vi "merFISH_define_buffer_probe_lists.vi"(4 "error in":errorcluster, 5 "Start acquisition":bool, 6 "Probe Refnum":refnum<vi>, 7 "Buffer Refnum":refnum<vi>) -> (0 "error out":errorcluster, 3 "Next task":T1)   [LabVIEW 2015]
uses:
  CONTROLS/Q_main_element.ctl
panel:
  in  "Remove probe":bool
  in  "Remove buffer":bool
  in  "stop":bool
  in  "merFISH probe":string
  in  "Valve #":i32
  in  "Add probe":bool
  in  "Buffer":string
  in  "Probe list":i32(listbox)=1
  in  "Buffer list":i32(listbox)=3
  in  "Valve #":i32
  in  "Add buffer":bool
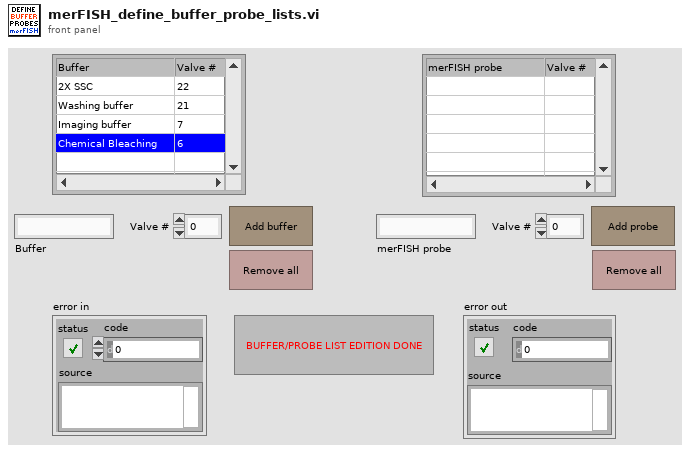
[diagram p1: front panel]
types:
  T1 = typedef "Q_main_element.ctl" = cluster{"variant":variant, "Instruction":enum16{"Main_idle", "Main_initialize", "Main_initialize_TDMS", "Main_initialize_Queue", "Main_error", "Main_DAQ_initialization_results", "Main_ASI_initialization_results", "Main_Piezo_initialization_results", "Main_Valve_initialization_results", "Main_Pump_initialization_results", "Main_CAMERA_initialization_results", "Main_FPGA_initialization_results", "Main_DAQ_error", "Main_ASI_error", "Main_Piezo_error", "Main_CAMERA_error", "Main_Valve_error", "Main_Pump_error", "Main_FPGA_error", "Main_start_acquiring", "Main_not_acquiring", "Main_acquiring", "Main_stop_acquiring", "Main_change_exposure", "Main_change_z_scan_parameters", "Main_define_ROI", "Main_define_mosaic", "Main_read_kinetic_time", "Main_cooler", "Main_read_temperature", "Main_save_XY", "Main_load_XY", "Main_discard_XY", "Main_move_to_XY", "Main_measure_QPD", "Main_autofocus_calibration", "Main_autofocus_initialization", "Main_autofocus_stop", "Main_save_PID", "Main_change_H_valve_position", "Main_two_way_valve", "Main_save_movie", "Main_init_single_scan", "Main_single_scan", "Main_stop_single_scan", "Main_merFISH_illumination_parameters", "Main_merFISH_buffer_probe_list", "Main_merFISH_injections_procedure", "Main_merFISH_save_setpoint", "Main_merFISH_DAPI_parameters", "Main_merFISH_Brightfield_parameters", "Main_merFISH_save_embryo_ROI", "Main_merFISH_init", "Main_merFISH_resume", "Main_merFISH_start_autofocus", "Main_merFISH_open_close_valve_merFISH", "Main_merFISH_open_close_valve_photobleaching", "Main_merFISH_hybridization", "Main_merFISH_move_to_ROI", "Main_merFISH_wait_stabilization", "Main_merFISH_move_to_REF", "Main_merFISH_scan", "Main_merFISH_photobleaching_injection", "Main_merFISH_photobleaching", "Main_merFISH_send_email", "Main_merFISH_close", "Main_STOP"}}
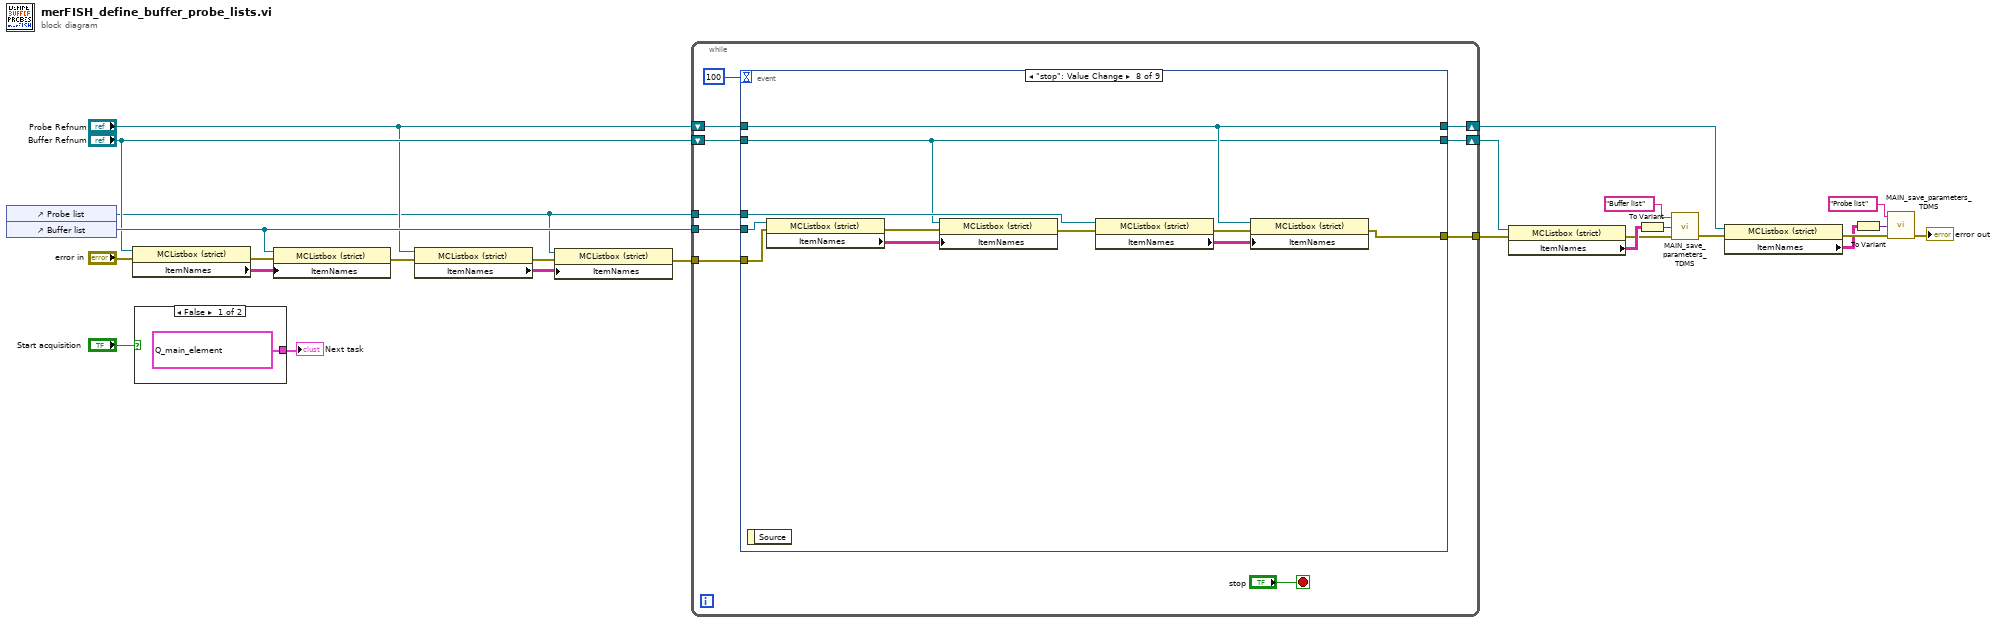
[diagram p0: block diagram]
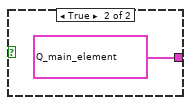
[diagram p2: hidden frame]
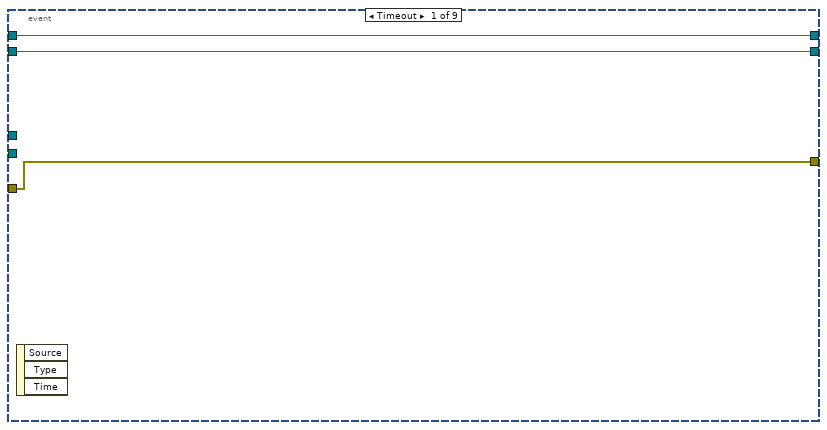
[diagram p3: hidden frame]
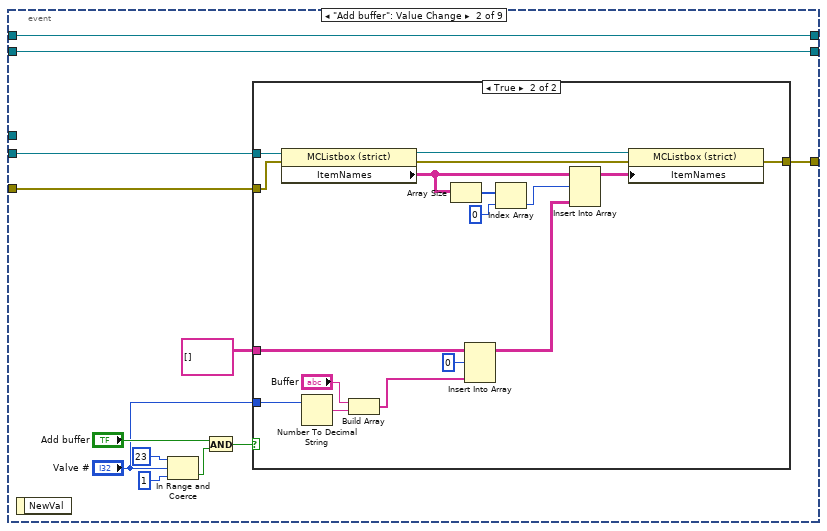
[diagram p4: hidden frame]
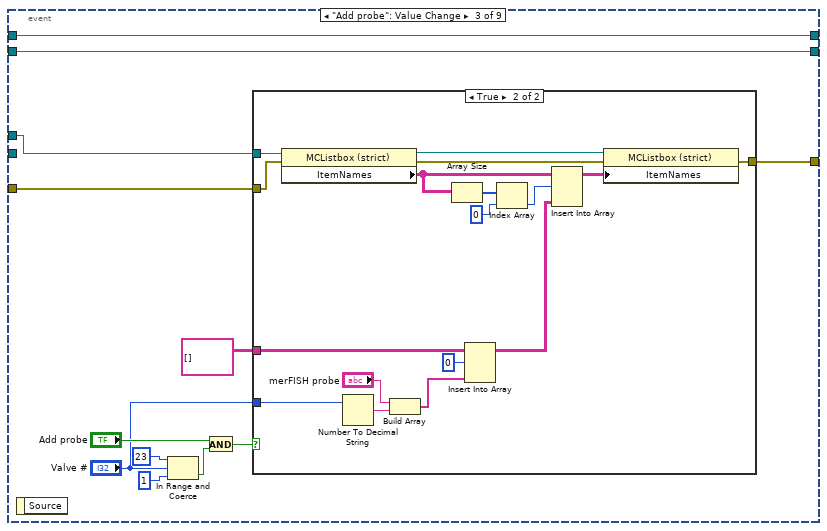
[diagram p6: hidden frame]
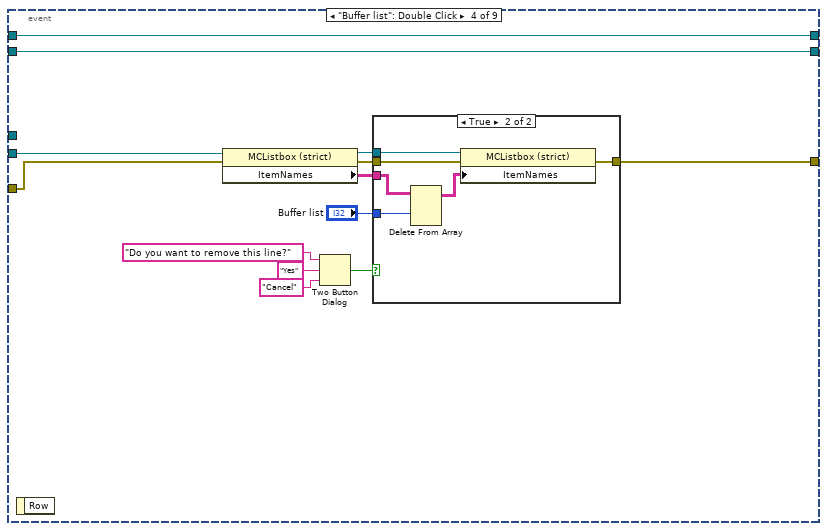
[diagram p8: hidden frame]
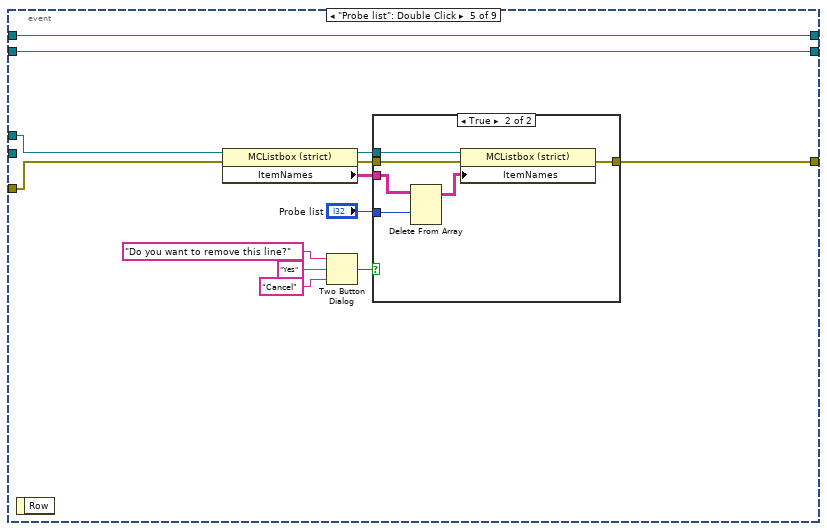
[diagram p10: hidden frame]
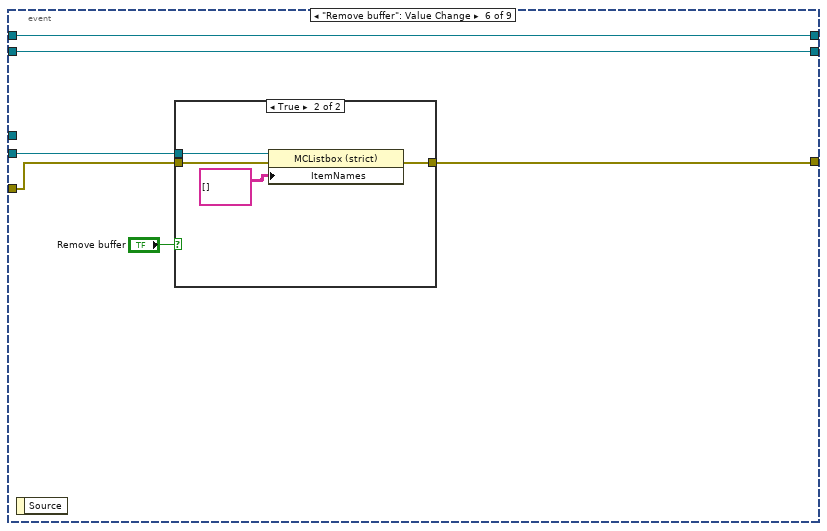
[diagram p12: hidden frame]
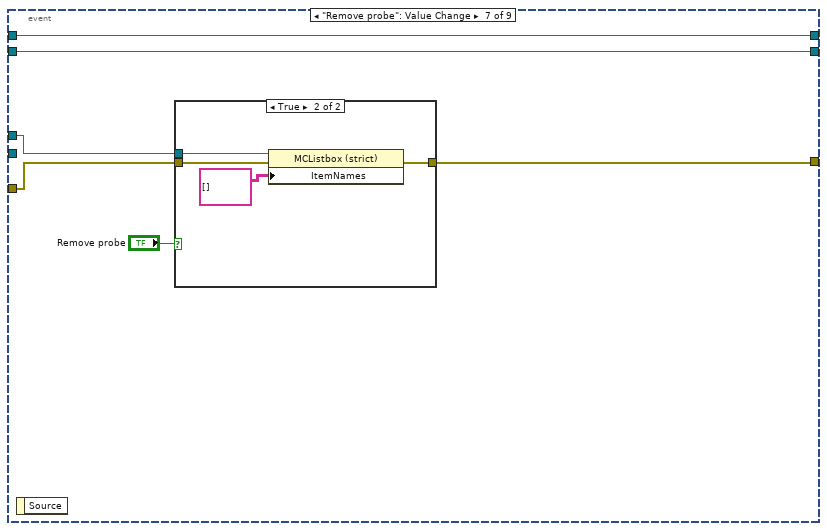
[diagram p14: hidden frame]
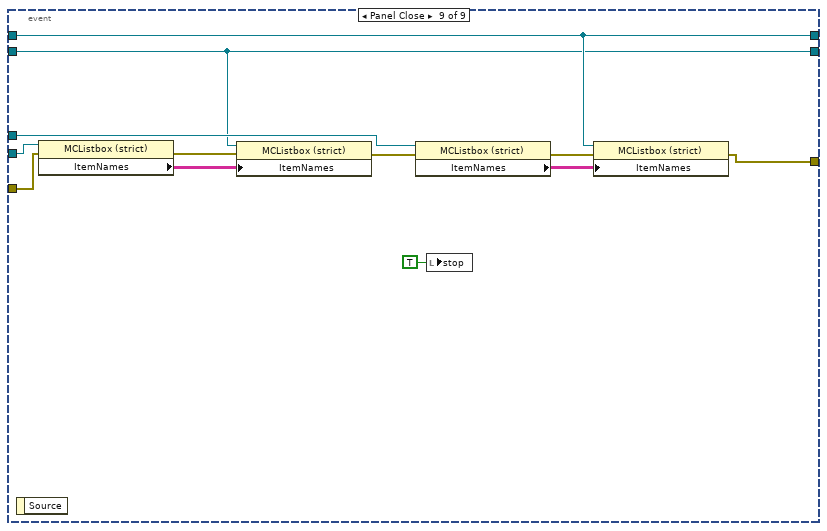
[diagram p16: hidden frame]
diagram:
  n1 = control-ref of="Probe list"() -> (w16:refnum<vi>)
  n2 = control-ref of="Buffer list"() -> (w26:refnum<vi>)
  n3 = property class="MCListbox (strict)"(reference="Buffer Refnum", error in="error in") -> (error out=w25:errorcluster, "ItemNames"=w23:string[][])  [unwired: 1 out]
  n4 = case shown="False" "Start acquisition" {
    tunnel: [T1 {"variant"=variant, "Instruction"=enum."Main_not_acquiring"} ("Q_main_element") T1 {"variant"=variant, "Instruction"=enum."Main_acquiring"} ("Q_main_element")] -> w1
    frame False {
    }
    frame True {
    }
  }
  "Next task" <- w1
  n5 = property class="MCListbox (strict)"(reference=w26, error in=w25, "ItemNames"=w23) -> (error out=w20:errorcluster)  [unwired: 1 out]
  n6 = property class="MCListbox (strict)"(reference="Probe Refnum", error in=w20) -> (error out=w21:errorcluster, "ItemNames"=w22:string[][])  [unwired: 1 out]
  n7 = property class="MCListbox (strict)"(reference=w16, error in=w21, "ItemNames"=w22) -> (error out=w18:errorcluster)  [unwired: 1 out]
  n8 = while {
    tunnel: w26 -> [w37]
    tunnel: w16 -> [w36]
    tunnel: [w35] -> w8
    tunnel: w18 -> [w31]
    shift-right: [w30] -> w3
    shift-left: "Probe Refnum" -> [w33]
    shift-right: [w29] -> w4
    shift-left: "Buffer Refnum" -> [w32]
    stop <- "stop" stop-if-true
    n9 = event shown="[7] \"stop\": Value Change" {
      selector: _ -> [_ _ _ _ _ _ _ _ _]
      dyn-events: _ -> [_ _ _ _ _ _ _ _ _]
      timeout: 100 -> [_ _ _ _ _ _ _ _ _]
      tunnel: [w41 w47 w79 w110 w130 w145 w158 w170 w182] -> w35
      tunnel: w37 -> [_ w46 _ w106 _ w146 _ w169 w181]
      tunnel: w36 -> [_ _ w77 _ w125 _ w156 w173 w185]
      tunnel: w33 -> [w40 w43 w73 w103 w123 w143 w154 w165 w176]
      tunnel: w32 -> [w39 w42 w72 w102 w122 w142 w153 w164 w175]
      tunnel: w31 -> [w41 w44 w74 w104 w124 w144 w155 w168 w180]
      tunnel: [w40 w43 w73 w103 w123 w143 w154 w165 w176] -> w30
      tunnel: [w39 w42 w72 w102 w122 w142 w153 w164 w175] -> w29
      event Timeout {
        n10 = event-data() -> ()  [unwired: 1 in, 3 out]
      }
      event "Add buffer": Value Change {
        n11 = event-data() -> ()  [unwired: 1 in, 1 out]
        n12 = In Range and Coerce(upper limit=23, x="Valve #", lower limit=1) -> (In Range?=w51:bool)  [unwired: 1 out]
        n13 = And(x="Add buffer", y=w51) -> (x .and. y?=w49:bool)
        n14 = case shown="True" w49 {
          tunnel: w46 -> [_ w71]
          tunnel: string[][] [] ("Item Names") -> [_ w70]
          tunnel: "Valve #" -> [_ w69]
          tunnel: [w54 w59] -> w47
          tunnel: w44 -> [w54 w58]
          frame False {
          }
          frame True {
            n15 = property class="MCListbox (strict)"(reference=w71, error in=w58) -> (reference out=w55:refnum<vi>, error out=w56:errorcluster, "ItemNames"=w57:string[][])
            n16 = Number To Decimal String(number=w69) -> (decimal integer string=w67:string)  [unwired: 1 in]
            n17 = Build Array("Buffer", w67) -> (w65:string[])
            n18 = Array Size(array=w57) -> (size(s)=w64:i32[])
            n19 = Insert Into Array(array=w70, index (row)=0, new element=w65) -> (w62:string[][])  [unwired: 1 in]
            n20 = Index Array(array=w64, index=0) -> (element=w61:i32)
            n21 = Insert Into Array(array=w57, index (row)=w61, new element=w62) -> (w60:string[][])  [unwired: 1 in]
            n22 = property class="MCListbox (strict)"(reference=w55, error in=w56, "ItemNames"=w60) -> (error out=w59:errorcluster)  [unwired: 1 out]
          }
        }
      }
      event "Add probe": Value Change {
        n23 = event-data() -> ()  [unwired: 1 in, 1 out]
        n24 = In Range and Coerce(upper limit=23, x="Valve #", lower limit=1) -> (In Range?=w81:bool)  [unwired: 1 out]
        n25 = And(x="Add probe", y=w81) -> (x .and. y?=w80:bool)
        n26 = case shown="True" w80 {
          tunnel: w77 -> [_ w101]
          tunnel: string[][] [] ("Item Names") -> [_ w100]
          tunnel: "Valve #" -> [_ w99]
          tunnel: [w84 w98] -> w79
          tunnel: w74 -> [w84 w88]
          frame False {
          }
          frame True {
            n27 = property class="MCListbox (strict)"(reference=w101, error in=w88) -> (reference out=w87:refnum<vi>, error out=w86:errorcluster, "ItemNames"=w85:string[][])
            n28 = Number To Decimal String(number=w99) -> (decimal integer string=w96:string)  [unwired: 1 in]
            n29 = Build Array("merFISH probe", w96) -> (w95:string[])
            n30 = Array Size(array=w85) -> (size(s)=w94:i32[])
            n31 = Insert Into Array(array=w100, index (row)=0, new element=w95) -> (w91:string[][])  [unwired: 1 in]
            n32 = Index Array(array=w94, index=0) -> (element=w92:i32)
            n33 = Insert Into Array(array=w85, index (row)=w92, new element=w91) -> (w90:string[][])  [unwired: 1 in]
            n34 = property class="MCListbox (strict)"(reference=w87, error in=w86, "ItemNames"=w90) -> (error out=w98:errorcluster)  [unwired: 1 out]
          }
        }
      }
      event "Buffer list": Double Click {
        n35 = event-data() -> ()  [unwired: 1 in, 1 out]
        n36 = property class="MCListbox (strict)"(reference=w106, error in=w104) -> (reference out=w109:refnum<vi>, error out=w108:errorcluster, "ItemNames"=w107:string[][])
        n37 = Two Button Dialog(message="Do you want to remove this line?", 1:"Cancel" ("F button name (\"Cancel\")"), 2:"Yes" ("T button name (\"OK\")")) -> (T button?=w111:bool)
        n38 = case shown="True" w111 {
          tunnel: w109 -> [_ w119]
          tunnel: [w115 w121] -> w110
          tunnel: w108 -> [w115 w120]
          tunnel: w107 -> [_ w117]
          tunnel: "Buffer list" -> [_ w118]
          frame False {
          }
          frame True {
            n39 = Delete From Array(array=w117, index (row)=w118) -> (array with subset deleted=w116:string[][])  [unwired: 2 in, 1 out]
            n40 = property class="MCListbox (strict)"(reference=w119, error in=w120, "ItemNames"=w116) -> (error out=w121:errorcluster)  [unwired: 1 out]
          }
        }
      }
      event "Probe list": Double Click {
        n41 = event-data() -> ()  [unwired: 1 in, 1 out]
        n42 = property class="MCListbox (strict)"(reference=w125, error in=w124) -> (reference out=w129:refnum<vi>, error out=w128:errorcluster, "ItemNames"=w127:string[][])
        n43 = Two Button Dialog(message="Do you want to remove this line?", 1:"Cancel" ("F button name (\"Cancel\")"), 2:"Yes" ("T button name (\"OK\")")) -> (T button?=w131:bool)
        n44 = case shown="True" w131 {
          tunnel: w129 -> [_ w139]
          tunnel: [w135 w141] -> w130
          tunnel: w128 -> [w135 w140]
          tunnel: w127 -> [_ w137]
          tunnel: "Probe list" -> [_ w138]
          frame False {
          }
          frame True {
            n45 = Delete From Array(array=w137, index (row)=w138) -> (array with subset deleted=w136:string[][])  [unwired: 2 in, 1 out]
            n46 = property class="MCListbox (strict)"(reference=w139, error in=w140, "ItemNames"=w136) -> (error out=w141:errorcluster)  [unwired: 1 out]
          }
        }
      }
      event "Remove buffer": Value Change {
        n47 = event-data() -> ()  [unwired: 1 in, 1 out]
        n48 = case shown="True" "Remove buffer" {
          tunnel: w146 -> [_ w152]
          tunnel: [w148 w151] -> w145
          tunnel: w144 -> [w148 w150]
          frame False {
          }
          frame True {
            n49 = property class="MCListbox (strict)"(reference=w152, error in=w150, "ItemNames"=string[][] [] ("array w/ subset deleted")) -> (error out=w151:errorcluster)  [unwired: 1 out]
          }
        }
      }
      event "Remove probe": Value Change {
        n50 = event-data() -> ()  [unwired: 1 in, 1 out]
        n51 = case shown="True" "Remove probe" {
          tunnel: w156 -> [_ w163]
          tunnel: [w159 w162] -> w158
          tunnel: w155 -> [w159 w161]
          frame False {
          }
          frame True {
            n52 = property class="MCListbox (strict)"(reference=w163, error in=w161, "ItemNames"=string[][] [] ("array w/ subset deleted")) -> (error out=w162:errorcluster)  [unwired: 1 out]
          }
        }
      }
      event "stop": Value Change {
        n53 = event-data() -> ()  [unwired: 1 in, 1 out]
        n54 = property class="MCListbox (strict)"(reference=w169, error in=w168) -> (error out=w167:errorcluster, "ItemNames"=w166:string[][])  [unwired: 1 out]
        n55 = property class="MCListbox (strict)"(reference=w164, error in=w167, "ItemNames"=w166) -> (error out=w174:errorcluster)  [unwired: 1 out]
        n56 = property class="MCListbox (strict)"(reference=w173, error in=w174) -> (error out=w171:errorcluster, "ItemNames"=w172:string[][])  [unwired: 1 out]
        n57 = property class="MCListbox (strict)"(reference=w165, error in=w171, "ItemNames"=w172) -> (error out=w170:errorcluster)  [unwired: 1 out]
      }
      event Panel Close {
        n58 = event-data() -> ()  [unwired: 1 in, 1 out]
        n59 = property class="MCListbox (strict)"(reference=w181, error in=w180) -> (error out=w179:errorcluster, "ItemNames"=w178:string[][])  [unwired: 1 out]
        n60 = property class="MCListbox (strict)"(reference=w175, error in=w179, "ItemNames"=w178) -> (error out=w186:errorcluster)  [unwired: 1 out]
        n61 = property class="MCListbox (strict)"(reference=w185, error in=w186) -> (error out=w183:errorcluster, "ItemNames"=w184:string[][])  [unwired: 1 out]
        n62 = local write "stop"(TRUE ("stop")) -> ()
        n63 = property class="MCListbox (strict)"(reference=w176, error in=w183, "ItemNames"=w184) -> (error out=w182:errorcluster)  [unwired: 1 out]
      }
    }
  }
  n64 = property class="MCListbox (strict)"(reference=w4, error in=w8) -> (error out=w9:errorcluster, "ItemNames"=w11:string[][])  [unwired: 1 out]
  n65 = To Variant(anything=w11) -> (Variant=w10:variant)
  n66 = call "MAIN_save_parameters_TDMS.vi"("error in"=w9, "Data"=w10, "Channel name"="Buffer list" ("group name")) -> ("error out"=w15:errorcluster)  [unwired: 2 in]
  n67 = property class="MCListbox (strict)"(reference=w3, error in=w15) -> (error out=w14:errorcluster, "ItemNames"=w12:string[][])  [unwired: 1 out]
  n68 = To Variant(anything=w12) -> (Variant=w13:variant)
  n69 = call "MAIN_save_parameters_TDMS.vi"("error in"=w14, "Data"=w13, "Channel name"="Probe list" ("group name")) -> ("error out"=→"error out":errorcluster)  [unwired: 2 in]
